vi "OP400ZP_OuCrash.vi"(2 "Booléen":bool, 3 "IN":T1=enum."Scan") -> (0 "out":T1=enum."Scan")   [LabVIEW 2020]
uses:
  OP400ZP_state.ctl
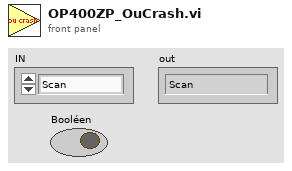
[diagram p1: front panel]
types:
  T1 = typedef "OP400ZP_state.ctl" = enum16{"Null", "Demarrage", "Init", "Scan", "Montage", "Conti", "Iso", "Vpack", "DataDyn", "Demontage", "Crash", "Next", "Sealing", "Comext"}
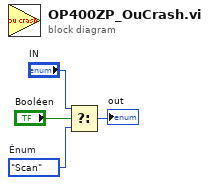
[diagram p0: block diagram]
diagram:
  w2 = OP400ZP_state."Scan"  # Énum
  n1 = Select(t="IN", s="Booléen", f=w2) -> (s? t:f=→"out":T1)
